vi "Sync Ch Set Sync Word.vi"(9 "pstSyncWord":T1, 10 "Channel":u8, 11 "devId":i32) -> (1 "pstSyncWord out":T1, 2 "devId out":i32, 3 "function return":i32)   [LabVIEW 2013, in "CHR34XXX.lvlib"]
doc: "DLL BOOL __stdcall CHR34XXX_Sync_Ch_LocalAddr(IN int devId,IN BYTE Channel,IN BYTE LocalAddr); DLL BOOL __stdcall CHR34XXX_Sync_Ch_SetCrc(IN int devId,IN BYTE Channel,IN BYTE CrcVal,IN BYTE CrcOrder); DLL BOOL __stdcall CHR34XXX_Sync_Ch_FrmId(IN int devId,IN BYTE Channel,IN WORD IdCnt,IN WORD IdPos,IN WORD IdOrder); DLL BOOL __stdcall CHR34XXX_Sync_Ch_MonitorEn(IN int devId,IN BYTE Channel,IN BOOL Enabled); DLL BOOL __stdcall CHR34XXX_Sync_Ch_TREdge(IN int devId,IN BYTE Channel,IN BYTE TxEdge,IN BYTE RxEdge); DLL BOOL __stdcall CHR34XXX_Sync_Ch_SetSyncWord(IN int devId,IN BYTE Channel,IN pCHRUART_SYNC_WORD_ST pstSyncWord);"
uses:
  CHR34XXX.lvlib
  CHR34XXX.dll
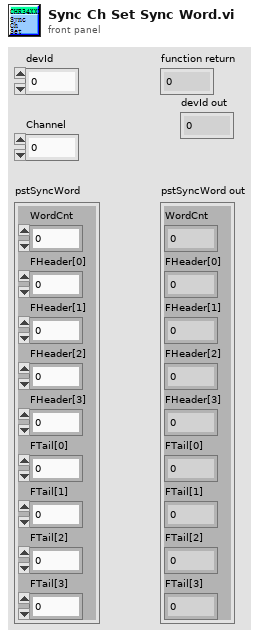
[diagram p1: front panel]
types:
  T1 = cluster{"WordCnt":u32, "FHeader[0]":u8, "FHeader[1]":u8, "FHeader[2]":u8, "FHeader[3]":u8, "FTail[0]":u8, "FTail[1]":u8, "FTail[2]":u8, "FTail[3]":u8}
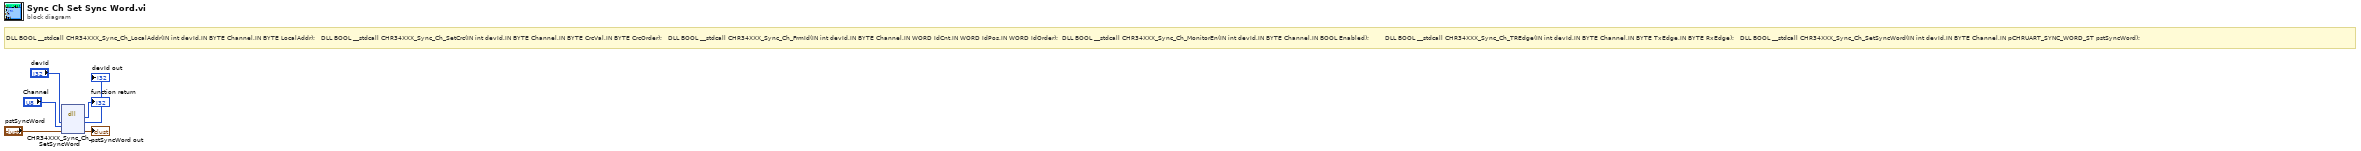
[diagram p0: block diagram]
diagram:
  # "DLL BOOL __stdcall CHR34XXX_Sync_Ch_LocalAddr(IN int devId,IN BYTE Channel,IN BYTE LocalAddr);   DLL BOOL __stdcall CHR34XXX_Sync_Ch_SetCrc(IN int devId,IN BYTE Channel,IN BYTE CrcVal,IN BYTE CrcOrder);   DLL BOOL __stdcall CHR34XXX_Sync_Ch_FrmId(IN int devId,IN BYTE Channel,IN WORD IdCnt,IN WORD IdPos,IN WORD IdOrder);  DLL BOOL __stdcall CHR34XXX_Sync_Ch_MonitorEn(IN int devId,IN BYTE Channel,IN BOOL Enabled);        DLL BOOL __stdcall CHR34XXX_Sync_Ch_TREdge(IN int devId,IN BYTE Channel,IN BYTE TxEdge,IN BYTE RxEdge);   DLL BOOL __stdcall CHR34XXX_Sync_Ch_SetSyncWord(IN int devId,IN BYTE Channel,IN pCHRUART_SYNC_WORD_ST pstSyncWord);"
  n1 = dll-call lib="C:/Users/Administrator/Desktop/CHR34XXX_lv/lv_lib/CHR34XXX.*" fn="CHR34XXX_Sync_Ch_SetSyncWord"("devId"="devId", "Channel"="Channel", "pstSyncWord"="pstSyncWord") -> ("返回类型"=→"function return":i32, "devId"=→"devId out":i32, "pstSyncWord"=→"pstSyncWord out":T1)  [unwired: 4 in, 2 out]
